vi "convert counts to eng.vi"(6 "Axis (1..4)":T1=1 items=["X"=1, "Y"=2, "Z"=3, "T"=4], 8 "error in (no error)":errorcluster, 9 "Position, counts":i32, 10 "All Positions, counts":i32[](array[numeric]), 11 "VXMx2 in":refnum<class "VXMx2.lvclass">) -> (0 "error out":errorcluster, 1 "Position, eng units":dbl, 2 "All Positions, eng units":dbl[](array[numeric]), 3 "VXMx2 out":refnum<class "VXMx2.lvclass">)   [LabVIEW 2018, in "VXMx2.lvclass"]
uses:
  VXMx2.lvclass
  <instrlib>/Velmex VXM/Public/VXM Axis.ctl
  VXMx2.lvclass/VXMx2.ctl
  <instrlib>/Velmex VXM/Velmex VXM.lvlib
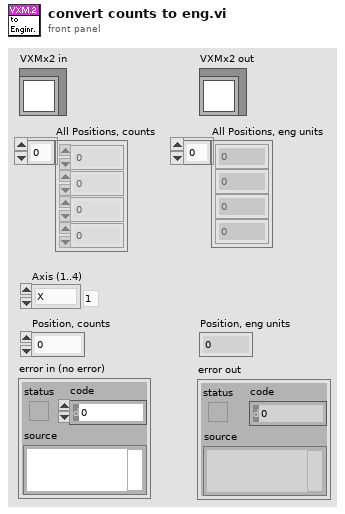
[diagram p1: front panel]
types:
  T1 = typedef "Velmex VXM.lvlib/VXM Axis.ctl" = u16
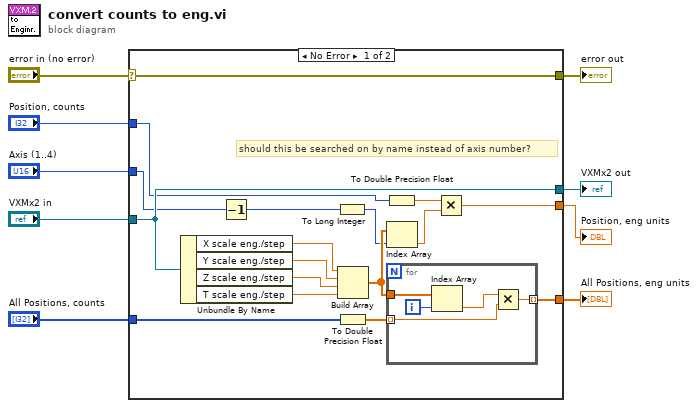
[diagram p0: block diagram]
diagram:
  n1 = case shown="No Error" "error in (no error)" {
    selector: "error in (no error)" -> [w26 w33]
    tunnel: [w26 w33] -> w1
    tunnel: [w25 w32] -> w4
    tunnel: "VXMx2 in" -> [w25 w32]
    tunnel: "All Positions, counts" -> [w20 _]
    tunnel: [w18 _] -> w8
    tunnel: "Axis (1..4)" -> [w16 _]
    tunnel: "Position, counts" -> [w13 _]
    tunnel: [w11 _] -> w5
    frame No Error {
      # "should this be searched on by name instead of axis number?"
      n2 = Unbundle By Name(w25) -> ("X scale eng./step"=w24:dbl, "Y scale eng./step"=w23:dbl, "Z scale eng./step"=w22:dbl, "T scale eng./step"=w21:dbl)
      n3 = Decrement(x=w16) -> (x-1=w15:T1)
      n4 = To Long Integer(number=w15) -> (32bit integer=w14:i32)
      n5 = Build Array(w24, w23, w22, w21) -> (w17:dbl[])
      n6 = To Double Precision Float(number=w20) -> (double precision float=w19:dbl[])
      n7 = To Double Precision Float(number=w13) -> (double precision float=w10:dbl)
      n8 = Index Array(array=w17, index=w14) -> (element=w12:dbl)
      n9 = for {
        tunnel: w17 -> [w29]
        tunnel: w19 -> [w27] mode=indexing
        tunnel: [w30] -> w18 mode=indexing
        i -> [w31]
        n10 = Index Array(array=w29, index=w31) -> (element=w28:dbl)
        n11 = Multiply(x=w28, y=w27) -> (x*y=w30:dbl)
      }
      n12 = Multiply(x=w10, y=w12) -> (x*y=w11:dbl)
    }
    frame Error {
    }
  }
  "error out" <- w1
  "VXMx2 out" <- w4
  "All Positions, eng units" <- w8
  "Position, eng units" <- w5
